vi "(SubVI) refine theme compare.vi"(1 "String in":string, 2 "Talent array":string[](array[string])) -> (0 "refine theme compare":string)   [LabVIEW 2022 SP3]
uses:
  <vilib>/Utility/error.llb/Trim Whitespace One-Sided.vi
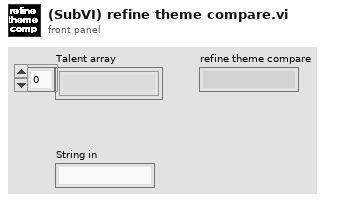
[diagram p1: front panel]
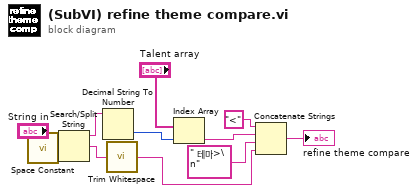
[diagram p0: block diagram]
diagram:
  n1 = call <vilib>:"Space Constant.vi"() -> ("String"=w1:string)
  n2 = Search/Split String(string="String in", search string/char (-)=w1) -> (substring before match=w3:string, match + rest of string=w6:string)  [unwired: 1 in, 1 out]
  n3 = Decimal String To Number(string=w3) -> (number=w5:i32)  [unwired: 2 in, 1 out]
  n4 = call <vilib>:"Trim Whitespace.vi"("string"=w6) -> ("trimmed string"=w10:string)  [unwired: 1 in]
  n5 = Index Array(array="Talent array", index=w5) -> (element=w8:string)
  n6 = Concatenate Strings("<", w8, " 테마>\n" ("string"), w10) -> (→"refine theme compare":string)
